vi "XIPIN_CORDIC_4_0.vi"   [LabVIEW 2017]
doc: "The Xilinx CORDIC LogiCORE is a module for generation of the generalized coordinate rotational digital computer (CORDIC) algorithm which iteratively solves trigonometric, hyperbolic and square root equations. The core is fully synchronous using a single clock. Options include parameterizable data width and control signals. The core supports either serial architecture for minimal area implementations, or parallel architecture for speed optimization. The core is delivered through the Xilinx CORE Generator System and integrates seamlessly with the Xilinx design flow.\n------------------------------------\n<b>Need License</b> : No"
uses:
  <vilib>/rvi/XilinxIP/XIPIN_XNode/niFpgaXIPIN.xnode
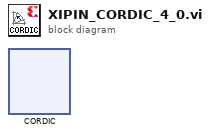
[diagram p0: block diagram]
diagram:
  n1 = xnode ("CORDIC")() -> ()
